vi "Array to JSON.vi"(7 "Include Name (T)":bool=TRUE, 8 "error in (no error)":errorcluster, 11 "Array":variant) -> (0 "error out":errorcluster, 3 "Array in JSON":string)   [LabVIEW 2011, in "LV JSON.lvlib"]
uses:
  LV JSON.lvlib
  <vilib>/Utility/VariantDataType/VariantType.lvlib
  <vilib>/Utility/error.llb/whitespace.ctl
panel:
  out "Name":string
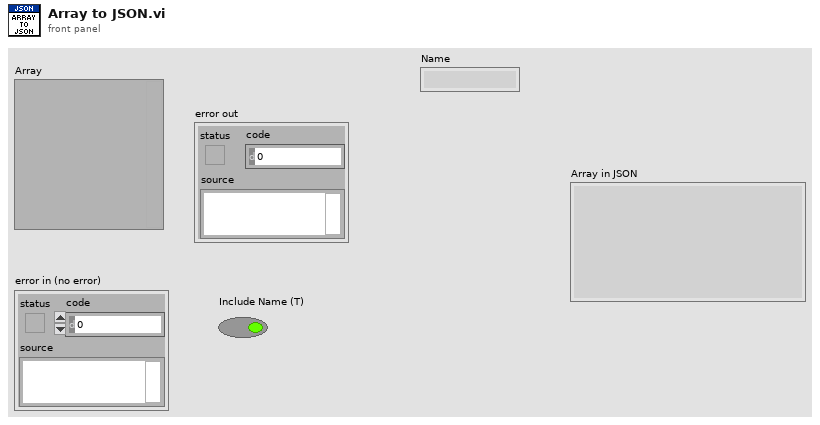
[diagram p1: front panel]
types:
  T1 = typedef "whitespace.ctl" = u16
  T2 = typedef "VariantType.lvlib/Type.ctl" = enum8{"Invalid Type", "Void", "I8", "I16", "I32", "I64", "U8", "U16", "U32", "U64", "Single Float", "Double Float", "Extended Float", "Single Complex", "Double Complex", "Extended Complex", "Enum U8", "Enum U16", "Enum U32", "Enum U64", "Single Float With Unit", "Double Float With Unit", "Extended Float With Unit", "Single Complex with Unit", "Double Complex with Unit", "Extended Complex with Unit", "Boolean", "String", "Path", "Picture", "Tag", "Array", "Cluster", "Variant", "LV Variant", "Waveform", "Timestamp", "Digital Waveform", "Digital Data", "ExpressData", "Refnum", "External Data", "VI", "Poly VI", "LabVIEW Class Instance", "Fixed Point"}
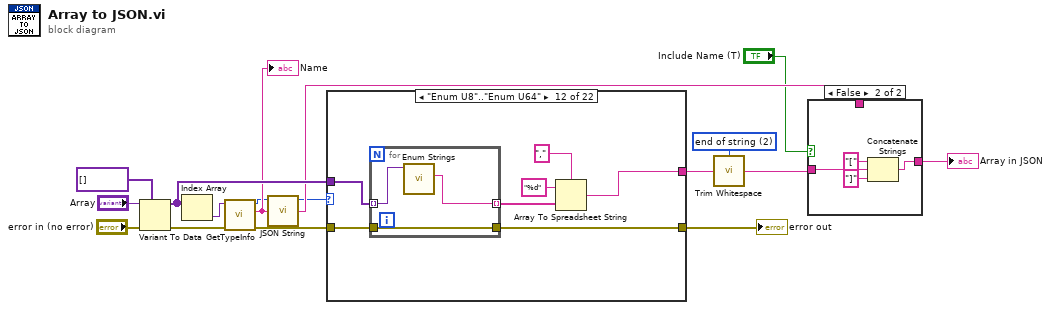
[diagram p0: block diagram]
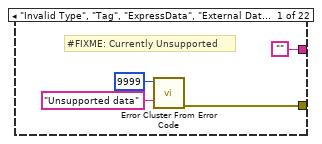
[diagram p2: hidden frame]
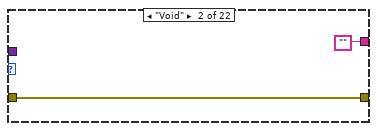
[diagram p3: hidden frame]
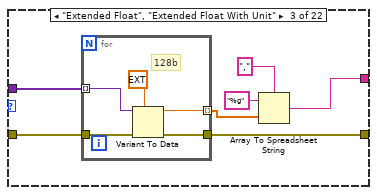
[diagram p4: hidden frame]
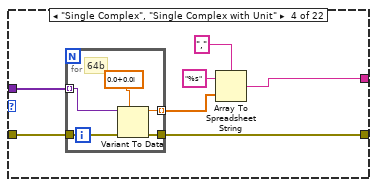
[diagram p5: hidden frame]
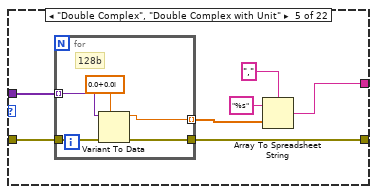
[diagram p6: hidden frame]
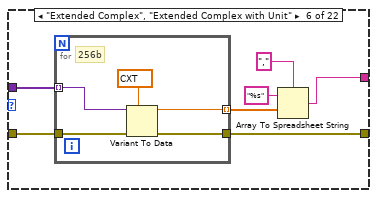
[diagram p7: hidden frame]
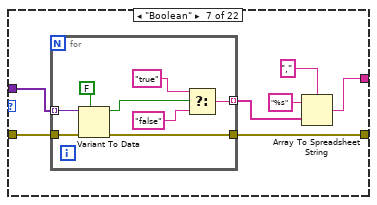
[diagram p8: hidden frame]
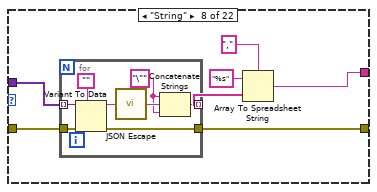
[diagram p9: hidden frame]
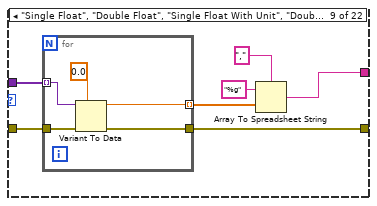
[diagram p10: hidden frame]
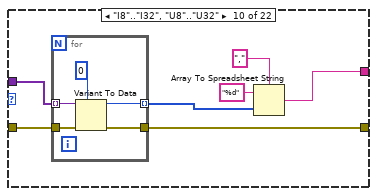
[diagram p11: hidden frame]
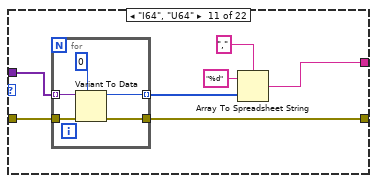
[diagram p12: hidden frame]
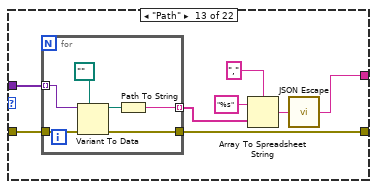
[diagram p13: hidden frame]
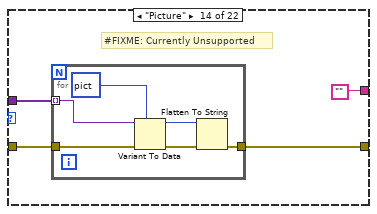
[diagram p14: hidden frame]
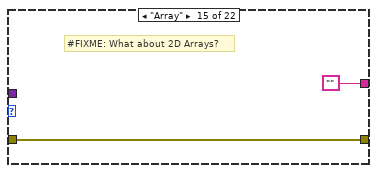
[diagram p15: hidden frame]
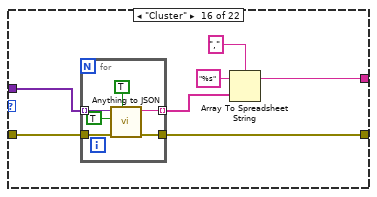
[diagram p16: hidden frame]
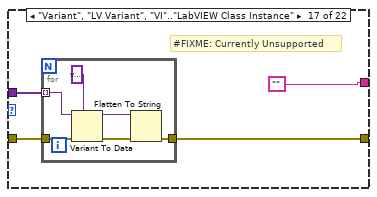
[diagram p17: hidden frame]
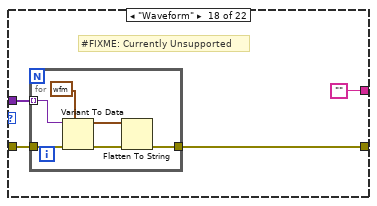
[diagram p18: hidden frame]
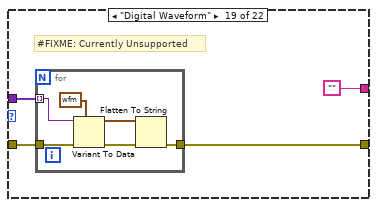
[diagram p19: hidden frame]
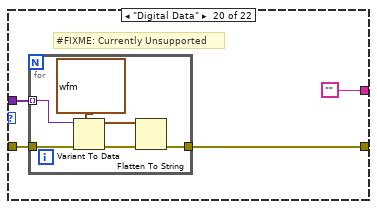
[diagram p20: hidden frame]
diagram:
  w10 = T1 2 items=["both", "start of string", "end of string"] ("location (both)")
  n1 = Variant To Data(error in="error in (no error)", type=variant[] [], Variant="Array") -> (data=w14:variant[], error out=w7:errorcluster)
  n2 = Index Array(array=w14) -> (element=w15:variant)  [unwired: 1 in]
  n3 = call <vilib>:"GetTypeInfo.vi"("error in (no error)"=w7, "Variant"=w15) -> ("error out"=w13:errorcluster, "Name"=w6:string, "Type Enum"=w2:T2)  [unwired: 5 in, 2 out]
  "Name" <- w6
  n4 = call "JSON String.vi"("in"=w6) -> ("out"=w5:string)
  n5 = case shown="\"Enum U8\"..\"Enum U64\"" w2 {
    tunnel: w14 -> [_ _ w28 w41 w52 w64 w76 w92 w107 w119 w131 w143 w152 w162 _ w179 w188 w198 w208 w218 w228 w238]
    tunnel: w13 -> [_ w22 w29 w40 w53 w65 w77 w91 w106 w118 w130 w142 w154 w164 w171 w178 w189 w199 w209 w219 w229 w237]
    tunnel: [w20 w22 w27 w39 w51 w63 w75 w90 w105 w117 w129 w141 w153 w163 w171 w177 w187 w197 w207 w217 w227 w239] -> w9
    tunnel: ["" "" w23 w35 w47 w59 w71 w86 w101 w114 w125 w137 w147 "" "" w176 "" "" "" "" "" ""] -> w12
    frame "Invalid Type", "Tag", "ExpressData", "External Data", Default {
      # "#FIXME: Currently Unsupported"
      n6 = call <vilib>:"Error Cluster From Error Code.vi"("error message (\"\")"="Unsupported data" ("error message (\"\")"), "error code (0)"=9999) -> ("error out"=w20:errorcluster)  [unwired: 7 in]
    }
    frame "Void" {
    }
    frame "Extended Float", "Extended Float With Unit" {
      n7 = for {
        tunnel: w28 -> [w32] mode=indexing
        tunnel: [w30] -> w26 mode=indexing
        tunnel: w29 -> [w34]
        tunnel: [w31] -> w27
        # "128b"
        n8 = Variant To Data(error in=w34, type=ext 0.0, Variant=w32) -> (data=w30:ext, error out=w31:errorcluster)
      }
      n9 = Array To Spreadsheet String(delimiter (Tab)=",", array=w26, 3:"%g" ("format string")) -> (spreadsheet string=w23:string)
    }
    frame "Single Complex", "Single Complex with Unit" {
      n10 = for {
        tunnel: w41 -> [w45] mode=indexing
        tunnel: w40 -> [w44]
        tunnel: [w43] -> w39
        tunnel: [w42] -> w36 mode=indexing
        # "64b"
        n11 = Variant To Data(error in=w44, type=csg 0.0+0.0i, Variant=w45) -> (data=w42:csg, error out=w43:errorcluster)
      }
      n12 = Array To Spreadsheet String(delimiter (Tab)=",", array=w36, 3:"%s" ("format string")) -> (spreadsheet string=w35:string)
    }
    frame "Double Complex", "Double Complex with Unit" {
      n13 = for {
        tunnel: w53 -> [w57]
        tunnel: w52 -> [w56] mode=indexing
        tunnel: [w55] -> w51
        tunnel: [w54] -> w48 mode=indexing
        # "128b"
        n14 = Variant To Data(error in=w57, type=cdb 0.0+0.0i, Variant=w56) -> (data=w54:cdb, error out=w55:errorcluster)
      }
      n15 = Array To Spreadsheet String(delimiter (Tab)=",", array=w48, 3:"%s" ("format string")) -> (spreadsheet string=w47:string)
    }
    frame "Extended Complex", "Extended Complex with Unit" {
      n16 = for {
        tunnel: w65 -> [w69]
        tunnel: w64 -> [w68] mode=indexing
        tunnel: [w67] -> w63
        tunnel: [w66] -> w60 mode=indexing
        # "256b"
        n17 = Variant To Data(error in=w69, type=cxt 0.0+0.0i, Variant=w68) -> (data=w66:cxt, error out=w67:errorcluster)
      }
      n18 = Array To Spreadsheet String(delimiter (Tab)=",", array=w60, 3:"%s" ("format string")) -> (spreadsheet string=w59:string)
    }
    frame "Boolean" {
      n19 = for {
        tunnel: w77 -> [w85]
        tunnel: w76 -> [w84] mode=indexing
        tunnel: [w82] -> w75
        tunnel: [w78] -> w72 mode=indexing
        n20 = Variant To Data(error in=w85, type=FALSE, Variant=w84) -> (data=w79:bool, error out=w82:errorcluster)
        n21 = Select(t="true", s=w79, f="false") -> (s? t:f=w78:string)
      }
      n22 = Array To Spreadsheet String(delimiter (Tab)=",", array=w72, 3:"%s" ("format string")) -> (spreadsheet string=w71:string)
    }
    frame "String" {
      n23 = for {
        tunnel: w92 -> [w100] mode=indexing
        tunnel: w91 -> [w99]
        tunnel: [w98] -> w90
        tunnel: [w94] -> w87 mode=indexing
        w93 = "\""
        n24 = Variant To Data(error in=w99, type="", Variant=w100) -> (data=w96:string, error out=w98:errorcluster)
        n25 = call "JSON Escape.vi"("JSON String"=w96) -> ("Escaped JSON String"=w95:string)
        n26 = Concatenate Strings(w93, w95, w93) -> (w94:string)
      }
      n27 = Array To Spreadsheet String(delimiter (Tab)=",", array=w87, 3:"%s" ("format string")) -> (spreadsheet string=w86:string)
    }
    frame "Single Float", "Double Float", "Single Float With Unit", "Double Float With Unit", "Fixed Point" {
      n28 = for {
        tunnel: w107 -> [w112] mode=indexing
        tunnel: w106 -> [w111]
        tunnel: [w110] -> w105
        tunnel: [w108] -> w102 mode=indexing
        n29 = Variant To Data(error in=w111, type=0.0, Variant=w112) -> (data=w108:dbl, error out=w110:errorcluster)
      }
      n30 = Array To Spreadsheet String(delimiter (Tab)=",", array=w102, 3:"%g" ("format string")) -> (spreadsheet string=w101:string)
    }
    frame "I8".."I32", "U8".."U32" {
      n31 = for {
        tunnel: w119 -> [w124] mode=indexing
        tunnel: w118 -> [w123]
        tunnel: [w122] -> w117
        tunnel: [w120] -> w113 mode=indexing
        n32 = Variant To Data(error in=w123, type=i8 0, Variant=w124) -> (data=w120:i8, error out=w122:errorcluster)
      }
      n33 = Array To Spreadsheet String(delimiter (Tab)=",", array=w113, 3:"%d" ("format string")) -> (spreadsheet string=w114:string)
    }
    frame "I64", "U64" {
      n34 = for {
        tunnel: w131 -> [w136] mode=indexing
        tunnel: w130 -> [w135]
        tunnel: [w134] -> w129
        tunnel: [w132] -> w126 mode=indexing
        n35 = Variant To Data(error in=w135, type=i64 0, Variant=w136) -> (data=w132:i64, error out=w134:errorcluster)
      }
      n36 = Array To Spreadsheet String(delimiter (Tab)=",", array=w126, 3:"%d" ("format string")) -> (spreadsheet string=w125:string)
    }
    frame "Enum U8".."Enum U64" {
      n37 = for {
        tunnel: w143 -> [w146] mode=indexing
        tunnel: w142 -> [w144]
        tunnel: [w144] -> w141
        tunnel: [w145] -> w138 mode=indexing
        n38 = call "Enum Strings.vi"("Enum"=w146) -> ("Selected item"=w145:string)  [unwired: 8 in, 2 out]
      }
      n39 = Array To Spreadsheet String(delimiter (Tab)=",", array=w138, 3:"%d" ("format string")) -> (spreadsheet string=w137:string)
    }
    frame "Path" {
      n40 = for {
        tunnel: w154 -> [w159]
        tunnel: [w158] -> w153
        tunnel: w152 -> [w157] mode=indexing
        tunnel: [w155] -> w149 mode=indexing
        n41 = Variant To Data(error in=w159, type=path "", Variant=w157) -> (data=w156:path, error out=w158:errorcluster)
        n42 = Path To String(path=w156) -> (string=w155:string)
      }
      n43 = Array To Spreadsheet String(delimiter (Tab)=",", array=w149, 3:"%s" ("format string")) -> (spreadsheet string=w148:string)
      n44 = call "JSON Escape.vi"("JSON String"=w148) -> ("Escaped JSON String"=w147:string)
    }
    frame "Picture" {
      # "#FIXME: Currently Unsupported"
      n45 = for {
        tunnel: w164 -> [w168]
        tunnel: [w167] -> w163
        tunnel: w162 -> [w166] mode=indexing
        n46 = Variant To Data(error in=w168, type=picture data[5B] ("empty picture"), Variant=w166) -> (data=w170:picture, error out=w169:errorcluster)
        n47 = Flatten To String(anything=w170, error in (no error)=w169) -> (error out=w167:errorcluster)  [unwired: 2 in, 2 out]
      }
    }
    frame "Array" {
      # "#FIXME: What about 2D Arrays?"
    }
    frame "Cluster" {
      n48 = for {
        tunnel: w179 -> [w185] mode=indexing
        tunnel: [w184] -> w175 mode=indexing
        tunnel: w178 -> [w183]
        tunnel: [w182] -> w177
        n49 = call "Anything to JSON.vi"("Nested? (F)"=TRUE, "error in (no error)"=w183, "Ignore Name? (F)"=TRUE, "Anything"=w185) -> ("error out"=w182:errorcluster, "JSON"=w184:string)  [unwired: 5 in, 1 out]
      }
      n50 = Array To Spreadsheet String(delimiter (Tab)=",", array=w175, 3:"%s" ("format string")) -> (spreadsheet string=w176:string)
    }
    frame "Variant", "LV Variant", "VI".."LabVIEW Class Instance" {
      # "#FIXME: Currently Unsupported"
      n51 = for {
        tunnel: w189 -> [w193]
        tunnel: w188 -> [w191] mode=indexing
        tunnel: [w190] -> w187
        n52 = Variant To Data(error in=w193, type=variant ("variant"), Variant=w191) -> (data=w195:variant, error out=w194:errorcluster)
        n53 = Flatten To String(anything=w195, error in (no error)=w194) -> (error out=w190:errorcluster)  [unwired: 2 in, 2 out]
      }
    }
    frame "Waveform" {
      # "#FIXME: Currently Unsupported"
      n54 = for {
        tunnel: w199 -> [w205]
        tunnel: w198 -> [w204] mode=indexing
        tunnel: [w200] -> w197
        n55 = Variant To Data(error in=w205, type=waveform(dbl) {"t0"=timestamp(0 s since 1904-01-01), "dt"=1.0, "Y"=[]} ("waveform"), Variant=w204) -> (data=w202:waveform(dbl), error out=w201:errorcluster)
        n56 = Flatten To String(anything=w202, error in (no error)=w201) -> (error out=w200:errorcluster)  [unwired: 2 in, 2 out]
      }
    }
    frame "Digital Waveform" {
      # "#FIXME: Currently Unsupported"
      n57 = for {
        tunnel: w209 -> [w213]
        tunnel: w208 -> [w212] mode=indexing
        tunnel: [w211] -> w207
        n58 = Variant To Data(error in=w213, type=digitalwaveform {"t0"=timestamp(0 s since 1904-01-01), "dt"=0.0, "Y"={"transitions"=[], "data"=[]}, "error"={"status"=FALSE, "code"=37421928, "source"=""}} ("digital waveform out"), Variant=w212) -> (data=w215:digitalwaveform, error out=w214:errorcluster)
        n59 = Flatten To String(anything=w215, error in (no error)=w214) -> (error out=w211:errorcluster)  [unwired: 2 in, 2 out]
      }
    }
    frame "Digital Data" {
      # "#FIXME: Currently Unsupported"
      n60 = for {
        tunnel: w219 -> [w223]
        tunnel: w218 -> [w222] mode=indexing
        tunnel: [w221] -> w217
        n61 = Variant To Data(error in=w223, type=digitaldata {"transitions"=[], "data"=[]} ("digital data"), Variant=w222) -> (data=w225:digitaldata, error out=w224:errorcluster)
        n62 = Flatten To String(anything=w225, error in (no error)=w224) -> (error out=w221:errorcluster)  [unwired: 2 in, 2 out]
      }
    }
    frame "Refnum" {
      # "#FIXME: Currently Unsupported"
      n63 = for {
        tunnel: w229 -> [w235]
        tunnel: w228 -> [w234] mode=indexing
        tunnel: [w231] -> w227
        n64 = Variant To Data(error in=w235, type=refnum<file> refnum ("refnum"), Variant=w234) -> (data=w230:refnum<file>, error out=w232:errorcluster)
        n65 = Flatten To String(anything=w230, error in (no error)=w232) -> (error out=w231:errorcluster)  [unwired: 2 in, 2 out]
      }
    }
    frame "Timestamp" {
      # "#FIXME: Currently Unsupported"
      n66 = for {
        tunnel: [w242] -> w239
        tunnel: w238 -> [w241] mode=indexing
        tunnel: w237 -> [w240]
        n67 = Variant To Data(error in=w240, type=timestamp(0 s since 1904-01-01) ("refnum"), Variant=w241) -> (data=w243:timestamp, error out=w244:errorcluster)
        n68 = Flatten To String(anything=w243, error in (no error)=w244) -> (error out=w242:errorcluster)  [unwired: 2 in, 2 out]
      }
    }
  }
  "error out" <- w9
  n69 = call <vilib>:"Trim Whitespace.vi"("string"=w12, "location (both)"=w10) -> ("trimmed string"=w1:string)
  n70 = case shown="False" "Include Name (T)" {
    tunnel: [w249 w253] -> w11
    tunnel: w1 -> [w248 w252]
    tunnel: w5 -> [w246 _]
    frame True {
      n71 = Concatenate Strings(w246, ":" ("string"), "[" ("string"), w248, "]" ("string")) -> (w249:string)
    }
    frame False {
      n72 = Concatenate Strings("[" ("string"), w252, "]" ("string")) -> (w253:string)
    }
  }
  "Array in JSON" <- w11
